vi "ADO Connection Get Data Types.vi"(8 "error in (no error)":errorcluster caption="错误输入（无错误）", 9 "file?":bool, 11 "Database Connection 输入":refnum<class "Database Connection.lvclass"> caption="DNL_LabVIEW Object in") -> (0 "error out":errorcluster caption="错误输出", 1 "database":enum16{"dBase", "Jet", "SQL Server", "Oracle"}(ring), 2 "data types":string[](array[string]), 3 "Database Connection 输出":refnum<class "Database Connection.lvclass"> caption="DNL_LabVIEW Object out")   [LabVIEW 2011, in "Database Connection.lvclass"]
uses:
  Database Connection.lvclass
  Database Connection.lvclass/Database Connection.ctl
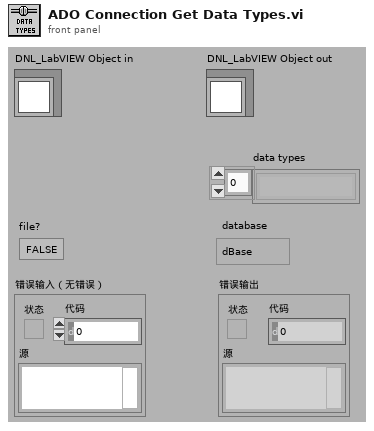
[diagram p1: front panel]
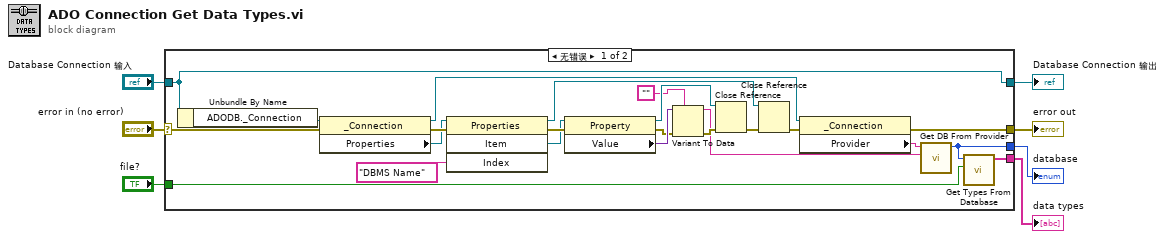
[diagram p0: block diagram]
diagram:
  n1 = case shown="无错误" "error in (no error)" {
    selector: "error in (no error)" -> [w14 w32]
    tunnel: [w9 w32] -> w6
    tunnel: [w30 w31] -> w4
    tunnel: "Database Connection 输入" -> [w30 w31]
    tunnel: "file?" -> [w11 _]
    tunnel: [w10 _] -> w2
    tunnel: [w8 _] -> w1
    frame No Error {
      n2 = Unbundle By Name(w30) -> ("ADODB._Connection"=w15:refnum<k7>)
      n3 = property class="_Connection"(reference=w15, error in=w14) -> (reference out=w28:refnum<k7>, error out=w21:errorcluster, "Properties"=w20:refnum<k7>)
      n4 = invoke class="Properties" method="Item"(reference=w20, error in=w21, "Index"="DBMS Name") -> (reference out=w22:refnum<k7>, error out=w24:errorcluster, "Item"=w23:refnum<k7>)  [unwired: 1 in, 1 out]
      n5 = property class="Property"(reference=w23, error in=w24) -> (reference out=w25:refnum<k7>, error out=w26:errorcluster, "Value"=w27:variant)
      n6 = Variant To Data(error in=w26, type="", Variant=w27) -> (data=w13:string, error out=w18:errorcluster)
      n7 = Close Reference(reference=w25, error in (no error)=w18) -> (error out=w19:errorcluster)
      n8 = Close Reference(reference=w22, error in (no error)=w19) -> (error out=w29:errorcluster)
      n9 = property class="_Connection"(reference=w28, error in=w29) -> (error out=w9:errorcluster, "Provider"=w12:string)  [unwired: 1 out]
      n10 = call "Get DB From Provider.vi"("DBMS Name"=w13, "Provider"=w12) -> ("database"=w10:enum16{"dBase", "Jet", "SQL Server", "Oracle"})  [unwired: 9 in]
      n11 = call "Get Types From Database.vi"("file?"=w11, "database"=w10) -> ("data types"=w8:string[])  [unwired: 8 in, 1 out]
    }
    frame Error {
    }
  }
  "error out" <- w6
  "Database Connection 输出" <- w4
  "database" <- w2
  "data types" <- w1
